vi "SubVI_SVM_train_Craik.vi"(4 "Max Passes":i32=15, 6 "C":dbl, 7 "Label Data":dbl[][](array[numeric]), 9 "Gamma":dbl, 10 "Linear or Gaussian":string, 11 "Training Data":dbl[][](array[numeric])) -> (0 "Alpha (idx)":dbl[][](array[numeric]), 1 "Label (idx)":dbl[][](array[numeric]), 2 "b":dbl, 3 "Training (idx)":dbl[][](array[numeric]), 5 "w":dbl[][](array[numeric]), 8 "Kernel Type":string)   [LabVIEW 2020]
uses:
  <vilib>/numeric/Random Number (Range) I64.vi
  <vilib>/Analysis/baseanly.llb/Real A x B.vi
  <vilib>/numeric/sub_Random U32.vi
  <vilib>/Analysis/Matrix/Numeric/Conversions/Matrix To Array - RM.vi
  <vilib>/Analysis/NI_AALBase.lvlib
  <vilib>/Analysis/Matrix/NI_Matrix.lvlib
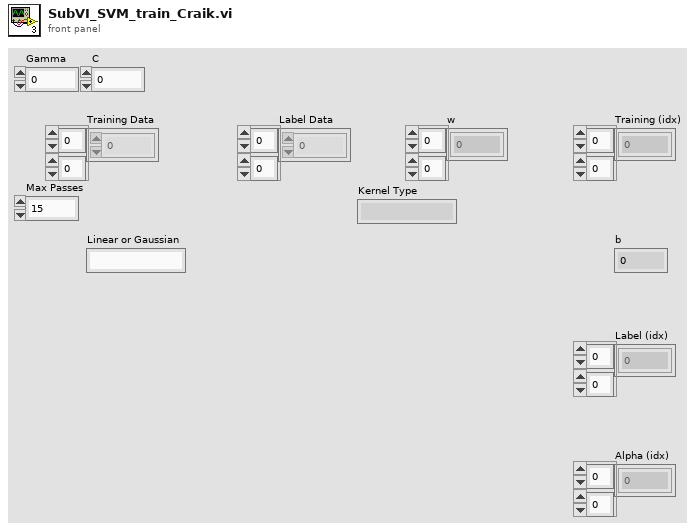
[diagram p1: front panel]
types:
  T1 = typedef "NI_Matrix.lvlib/RealMatrix.ctl" = dbl[][]
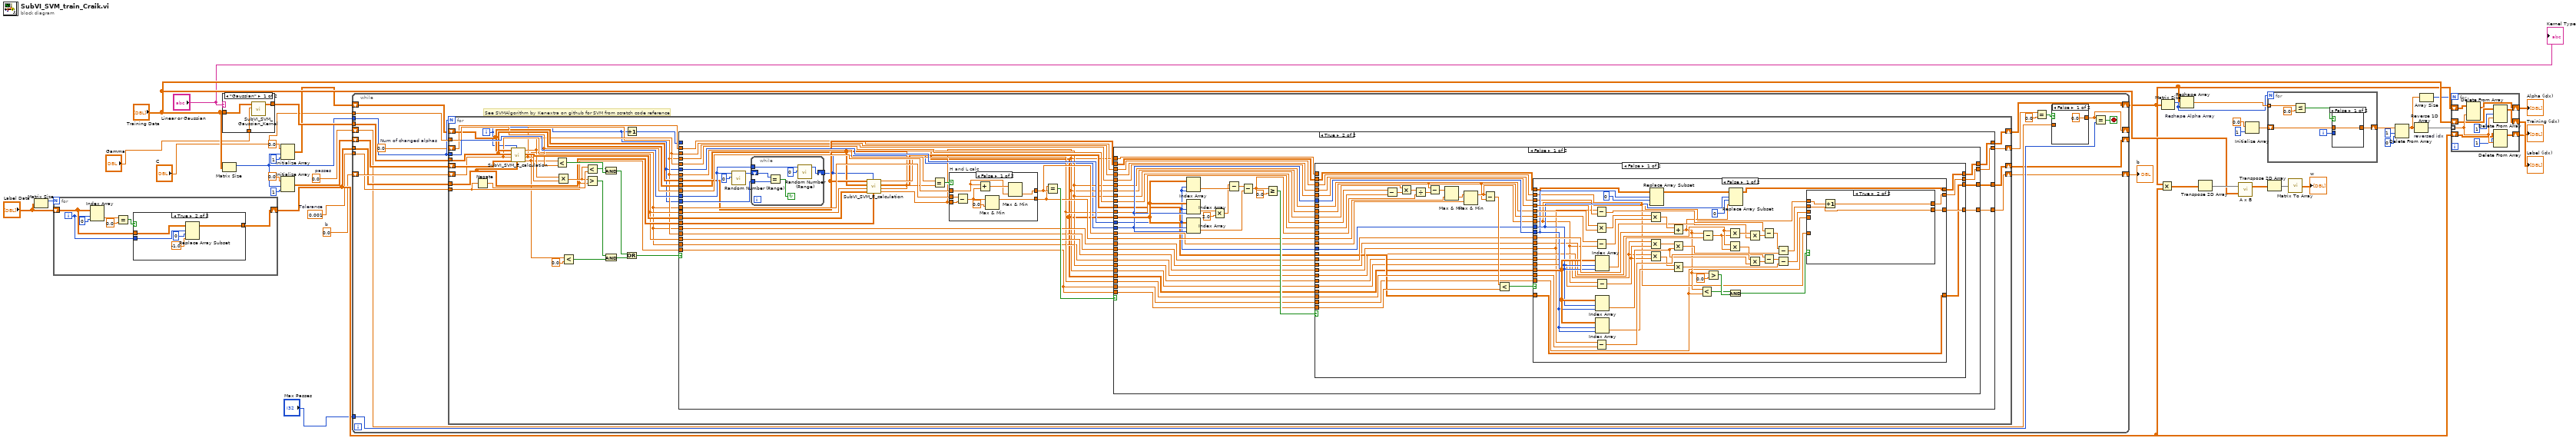
[diagram p0: block diagram]
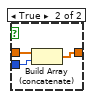
[diagram p2: hidden frame]
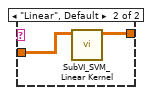
[diagram p3: hidden frame]
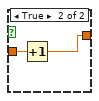
[diagram p4: hidden frame]
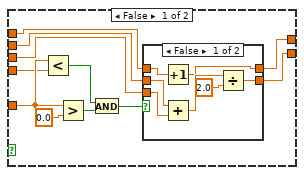
[diagram p6: hidden frame]
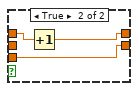
[diagram p7: hidden frame]
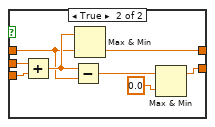
[diagram p11: hidden frame]
diagram:
  w4 = 0.001  # Tolerance
  w13 = 0.0  # passes
  w10 = 0.0  # b
  n1 = Matrix Size(0:"Label Data") -> (1:w5:i32)  [unwired: 1 out]
  n2 = for {
    N: w5 -> [_]
    shift-right: [w41] -> w40
    shift-left: "Label Data" -> [w43]
    i -> [w42]
    n3 = Index Array(array=w43, index (row)=w42, index (col)=0 ("disabled index (col)")) -> (element=w46:dbl)
    n4 = Equal?(x=w46, y=0.0) -> (x = y?=w47:bool)
    n5 = case shown="True" w47 {
      tunnel: w43 -> [w48 w53]
      tunnel: w42 -> [_ w52]
      tunnel: [w48 w49] -> w41
      frame False {
      }
      frame True {
        n6 = Replace Array Subset(array=w53, new element=-1.0 ("new element/subarray"), index (row)=w52, index (col)=0 ("disabled index (col)")) -> (w49:dbl[][])
      }
    }
  }
  n7 = case shown="\"Gaussian\"" "Linear or Gaussian" {
    tunnel: "Training Data" -> [w56 w58]
    tunnel: [w55 w57] -> w16
    tunnel: "Gamma" -> [w54 _]
    frame "Gaussian" {
      n8 = call "SubVI_SVM_Gaussian_Kernel.vi"("sigma"=w54, "X"=w56) -> ("K"=w55:dbl[][])  [unwired: 9 in]
    }
    frame "Linear", Default {
      n9 = call "SubVI_SVM_Linear Kernel.vi"("X"=w58) -> ("K"=w57:T1)  [unwired: 10 in]
    }
  }
  n10 = Matrix Size(0:"Training Data") -> (1:w12:i32)  [unwired: 1 out]
  n11 = Initialize Array(0.0 ("element"), w12, 1 ("dimension size")) -> (w14:dbl[][])
  n12 = Initialize Array(0.0 ("element"), w12, 1 ("dimension size")) -> (w11:dbl[][])
  n13 = while {
    tunnel: w40 -> [w76]
    tunnel: w4 -> [w74]
    tunnel: "C" -> [w73]
    tunnel: w12 -> [w72]
    shift-right: [w64] -> _
    shift-left: w13 -> [w66]
    tunnel: "Max Passes" -> [w63]
    shift-right: [w61] -> _
    shift-left: w11 -> [w75]
    tunnel: w16 -> [w70]
    shift-right: [w71] -> w32
    shift-left: w14 -> [w60]
    shift-right: [w59] -> w15
    shift-left: w10 -> [w77]
    stop <- w62 stop-if-true
    w69 = 0.0  # Num of changed alphas
    # "See SVMAlgorithm by Kenextra on github for SVM from scratch code reference"
    n14 = for {
      N: w72 -> [_]
      tunnel: w70 -> [w97]
      shift-right: [w91] -> w71
      shift-left: w60 -> [w92]
      tunnel: w76 -> [w95]
      shift-right: [w87] -> w61
      shift-left: w75 -> [w109]
      tunnel: w74 -> [w93]
      tunnel: w73 -> [w94]
      tunnel: w72 -> [w98]
      shift-right: [w89] -> w59
      shift-left: w77 -> [w90]
      shift-right: [w83] -> w68
      shift-left: w69 -> [w84]
      i -> [w82]
      n15 = Negate(x=w93) -> (-x=w108:dbl)
      n16 = call "SubVI_SVM_E_calculation.vi"("Y"=w95, "Index"=w82, "E"=w109, "b"=w90, "K"=w97, "Alphas"=w92) -> ("alpha[index]"=w85:dbl, "y[index]"=w86:dbl, "E"=w96:T1, "E[index]"=w88:dbl)  [unwired: 2 in]
      n17 = Less?(x=w85, y=w94) -> (x < y?=w107:bool)
      n18 = Multiply(x=w88, y=w86) -> (x*y=w105:dbl)
      n19 = Less?(x=w85, y=0.0) -> (x < y?=w102:bool)
      n20 = Less?(x=w105, y=w108) -> (x < y?=w106:bool)
      n21 = Greater?(x=w105, y=w93) -> (0:w104:bool)
      n22 = And(x=w106, y=w107) -> (x .and. y?=w100:bool)
      n23 = And(x=w104, y=w102) -> (x .and. y?=w101:bool)
      n24 = Or(x=w100, y=w101) -> (x .or. y?=w99:bool)
      n25 = Increment(x=w82) -> (x+1=w81:i32)
      n26 = case shown="True" w99 {
        tunnel: w98 -> [_ w146]
        tunnel: w82 -> [_ w147]
        tunnel: w92 -> [w113 w135]
        tunnel: w97 -> [_ w119]
        tunnel: w90 -> [_ w144]
        tunnel: w96 -> [w111 w143]
        tunnel: w95 -> [_ w142]
        tunnel: w86 -> [_ w141]
        tunnel: w85 -> [_ w139]
        tunnel: w94 -> [_ w138]
        tunnel: w82 -> [_ w136]
        tunnel: w88 -> [_ w134]
        tunnel: w93 -> [_ w118]
        tunnel: w85 -> [_ w131]
        tunnel: w86 -> [_ w130]
        tunnel: [w113 w129] -> w91
        tunnel: w90 -> [w112 w128]
        tunnel: [w112 w114] -> w89
        tunnel: w88 -> [_ w127]
        tunnel: [w111 w124] -> w87
        tunnel: w86 -> [_ w123]
        tunnel: w85 -> [_ w121]
        tunnel: w84 -> [w110 w117]
        tunnel: [w110 w116] -> w83
        tunnel: w81 -> [_ _]
        frame False {
        }
        frame True {
          n27 = call-poly <vilib>:"Random Number (Range).vi"("lower bound (-100)"=i64 0, "upper bound (100)"=w146) -> ("number"=w148:i64)  [unwired: 9 in]
          n28 = while {
            shift-right: [w330] -> w115
            shift-left: w148 -> [w334]
            tunnel: w147 -> [w333]
            tunnel: w146 -> [w331]
            stop <- w332 continue-if-true
            n29 = Equal?(x=w334, y=w333) -> (x = y?=w332:bool)
            n30 = call-poly <vilib>:"Random Number (Range).vi"("lower bound (-100)"=i64 0, "upper bound (100)"=w331) -> ("number"=w330:i64)  [unwired: 9 in]
          }
          n31 = call "SubVI_SVM_E_calculation.vi"("Y"=w142, "Index"=w115, "E"=w143, "b"=w144, "K"=w119, "Alphas"=w135) -> ("alpha[index]"=w120:dbl, "y[index]"=w122:dbl, "E"=w125:T1, "E[index]"=w126:dbl)  [unwired: 2 in]
          n32 = Equal?(x=w141, y=w122) -> (x = y?=w140:bool)
          n33 = case "H and L calc" shown="False" w140 {
            tunnel: w139 -> [w320 w328]
            tunnel: w120 -> [w319 w327]
            tunnel: w138 -> [w314 w322]
            tunnel: [w317 w324] -> w132
            tunnel: [w313 w321] -> w133
            frame False {
              n34 = Subtract(x=w320, y=w319) -> (x-y=w316:dbl)
              n35 = Add(x=w314, y=w316) -> (x+y=w315:dbl)
              n36 = Max & Min(x=w316, y=0.0) -> (max(x,y)=w317:dbl)  [unwired: 1 out]
              n37 = Max & Min(x=w315, y=w314) -> (min(x,y)=w313:dbl)  [unwired: 1 out]
            }
            frame True {
              n38 = Add(x=w328, y=w327) -> (x+y=w323:dbl)
              n39 = Subtract(x=w323, y=w322) -> (x-y=w326:dbl)
              n40 = Max & Min(x=w323, y=w322) -> (min(x,y)=w321:dbl)  [unwired: 1 out]
              n41 = Max & Min(x=w326, y=0.0) -> (max(x,y)=w324:dbl)  [unwired: 1 out]
            }
          }
          n42 = Equal?(x=w132, y=w133) -> (x = y?=w137:bool)
          n43 = case shown="False" w137 {
            tunnel: w119 -> [w187 _]
            tunnel: w136 -> [w168 _]
            tunnel: w115 -> [w180 _]
            tunnel: w135 -> [w181 w312]
            tunnel: w120 -> [w179 _]
            tunnel: w122 -> [w178 _]
            tunnel: w126 -> [w177 _]
            tunnel: w134 -> [w176 _]
            tunnel: w133 -> [w175 _]
            tunnel: w132 -> [w174 _]
            tunnel: w120 -> [w173 _]
            tunnel: w118 -> [w172 _]
            tunnel: w131 -> [w171 _]
            tunnel: w130 -> [w170 _]
            tunnel: w122 -> [w169 _]
            tunnel: [w167 w312] -> w129
            tunnel: w128 -> [w162 w311]
            tunnel: [w161 w311] -> w114
            tunnel: w127 -> [w160 _]
            tunnel: w126 -> [w159 _]
            tunnel: w125 -> [w158 w310]
            tunnel: [w157 w310] -> w124
            tunnel: w123 -> [w156 _]
            tunnel: w122 -> [w155 _]
            tunnel: w121 -> [w154 _]
            tunnel: w120 -> [w153 _]
            tunnel: w119 -> [w152 _]
            tunnel: w118 -> [w151 _]
            tunnel: w117 -> [w150 w309]
            tunnel: [w149 w309] -> w116
            frame False {
              n44 = Index Array(array=w187, index (row)=w168, index (col)=w168) -> (element=w186:dbl)
              n45 = Index Array(array=w187, index (row)=w168, index (col)=w180) -> (element=w166:dbl)
              n46 = Index Array(array=w187, index (row)=w180, index (col)=w180) -> (element=w184:dbl)
              n47 = Multiply(x=w166, y=2.0) -> (x*y=w164:dbl)
              n48 = Subtract(x=w164, y=w186) -> (x-y=w185:dbl)
              n49 = Subtract(x=w185, y=w184) -> (x-y=w163:dbl)
              n50 = Greater Or Equal?(x=w163, y=0.0) -> (x >= y?=w182:bool)
              n51 = case shown="False" w182 {
                tunnel: w181 -> [w224 w308]
                tunnel: w180 -> [w223 _]
                tunnel: w179 -> [_ _]
                tunnel: w178 -> [w220 _]
                tunnel: w177 -> [w221 _]
                tunnel: w176 -> [w222 _]
                tunnel: w163 -> [w217 _]
                tunnel: w175 -> [w216 _]
                tunnel: w174 -> [w214 _]
                tunnel: w173 -> [w204 _]
                tunnel: w172 -> [w212 _]
                tunnel: w171 -> [w209 _]
                tunnel: w170 -> [w208 _]
                tunnel: w169 -> [w207 _]
                tunnel: w168 -> [w206 _]
                tunnel: [w205 w308] -> w167
                tunnel: w162 -> [w201 w307]
                tunnel: [w200 w307] -> w161
                tunnel: w160 -> [w199 _]
                tunnel: w159 -> [w198 _]
                tunnel: w158 -> [w197 w306]
                tunnel: [w196 w306] -> w157
                tunnel: w156 -> [w195 _]
                tunnel: w155 -> [w194 _]
                tunnel: w154 -> [w193 _]
                tunnel: w153 -> [w192 _]
                tunnel: w152 -> [w191 _]
                tunnel: w151 -> [w190 _]
                tunnel: w150 -> [w189 w305]
                tunnel: [w188 w305] -> w149
                frame False {
                  n52 = Subtract(x=w222, y=w221) -> (x-y=w219:dbl)
                  n53 = Multiply(x=w220, y=w219) -> (x*y=w218:dbl)
                  n54 = Divide(x=w218, y=w217) -> (x/y=w203:dbl)
                  n55 = Subtract(x=w204, y=w203) -> (x-y=w202:dbl)
                  n56 = Max & Min(x=w202, y=w216) -> (min(x,y)=w215:dbl)  [unwired: 1 out]
                  n57 = Max & Min(x=w215, y=w214) -> (max(x,y)=w210:dbl)  [unwired: 1 out]
                  n58 = Subtract(x=w210, y=w204) -> (x-y=w213:dbl)
                  n59 = Less?(x=w213, y=w212) -> (x < y?=w211:bool)
                  n60 = case shown="False" w211 {
                    tunnel: w224 -> [w276 w304]
                    tunnel: w223 -> [w261 _]
                    tunnel: [w272 w304] -> w205
                    tunnel: w210 -> [w229 _]
                    tunnel: w209 -> [w266 _]
                    tunnel: w204 -> [w274 _]
                    tunnel: w208 -> [w270 _]
                    tunnel: w207 -> [w269 _]
                    tunnel: w206 -> [w262 _]
                    tunnel: w201 -> [w244 w303]
                    tunnel: [w230 w303] -> w200
                    tunnel: w199 -> [w257 _]
                    tunnel: w198 -> [w243 _]
                    tunnel: [w264 w302] -> w196
                    tunnel: w197 -> [w264 w302]
                    tunnel: w195 -> [w242 _]
                    tunnel: w194 -> [w238 _]
                    tunnel: w193 -> [w260 _]
                    tunnel: w192 -> [w254 _]
                    tunnel: w191 -> [w263 _]
                    tunnel: w190 -> [w227 _]
                    tunnel: w189 -> [w226 w301]
                    tunnel: [w225 w301] -> w188
                    frame False {
                      n61 = Subtract(x=w244, y=w257) -> (x-y=w256:dbl)
                      n62 = Multiply(x=w270, y=w269) -> (x*y=w267:dbl)
                      n63 = Subtract(x=w274, y=w229) -> (x-y=w268:dbl)
                      n64 = Subtract(x=w244, y=w243) -> (x-y=w249:dbl)
                      n65 = Subtract(x=w229, y=w254) -> (x-y=w239:dbl)
                      n66 = Index Array(array=w263, index (row)=w262, index (col)=w262) -> (element=w258:dbl)
                      n67 = Index Array(array=w263, index (row)=w262, index (col)=w261) -> (element=w240:dbl)
                      n68 = Index Array(array=w263, index (row)=w261, index (col)=w261) -> (element=w237:dbl)
                      n69 = Multiply(x=w267, y=w268) -> (x*y=w265:dbl)
                      n70 = Multiply(x=w238, y=w239) -> (x*y=w253:dbl)
                      n71 = Multiply(x=w238, y=w239) -> (x*y=w247:dbl)
                      n72 = Replace Array Subset(array=w276, new element=w229, index (row)=w261, index (col)=0 ("disabled index (col)")) -> (w273:dbl[][])
                      n73 = Add(x=w265, y=w266) -> (x+y=w235:dbl)
                      n74 = Multiply(x=w253, y=w240) -> (x*y=w251:dbl)
                      n75 = Multiply(x=w247, y=w237) -> (x*y=w245:dbl)
                      n76 = Less?(x=w235, y=w227) -> (x < y?=w233:bool)
                      n77 = Subtract(x=w235, y=w260) -> (x-y=w241:dbl)
                      n78 = Greater?(x=w235, y=0.0) -> (0:w234:bool)
                      n79 = Multiply(x=w242, y=w241) -> (x*y=w259:dbl)
                      n80 = Multiply(x=w242, y=w241) -> (x*y=w250:dbl)
                      n81 = And(x=w233, y=w234) -> (x .and. y?=w232:bool)
                      n82 = Replace Array Subset(array=w273, new element=w235, index (row)=w262, index (col)=0 ("disabled index (col)")) -> (w272:dbl[][])
                      n83 = Multiply(x=w259, y=w258) -> (x*y=w255:dbl)
                      n84 = Multiply(x=w250, y=w240) -> (x*y=w248:dbl)
                      n85 = Subtract(x=w256, y=w255) -> (x-y=w252:dbl)
                      n86 = Subtract(x=w249, y=w248) -> (x-y=w246:dbl)
                      n87 = Subtract(x=w252, y=w251) -> (x-y=w231:dbl)
                      n88 = Subtract(x=w246, y=w245) -> (x-y=w228:dbl)
                      n89 = case shown="True" w232 {
                        tunnel: w231 -> [w280 w300]
                        tunnel: [w281 w300] -> w230
                        tunnel: w229 -> [w284 _]
                        tunnel: w228 -> [w282 _]
                        tunnel: w227 -> [w279 _]
                        tunnel: w226 -> [w278 w299]
                        tunnel: [w277 w298] -> w225
                        frame False {
                          n90 = Less?(x=w284, y=w279) -> (x < y?=w285:bool)
                          n91 = Greater?(x=w284, y=0.0) -> (0:w286:bool)
                          n92 = And(x=w285, y=w286) -> (x .and. y?=w283:bool)
                          n93 = case shown="False" w283 {
                            tunnel: w282 -> [w293 w297]
                            tunnel: [w290 w297] -> w281
                            tunnel: w280 -> [w294 _]
                            tunnel: w278 -> [w289 w296]
                            tunnel: [w288 w295] -> w277
                            frame False {
                              n94 = Increment(x=w289) -> (x+1=w288:dbl)
                              n95 = Add(x=w294, y=w293) -> (x+y=w292:dbl)
                              n96 = Divide(x=w292, y=2.0) -> (x/y=w290:dbl)
                            }
                            frame True {
                              n97 = Increment(x=w296) -> (x+1=w295:dbl)
                            }
                          }
                        }
                        frame True {
                          n98 = Increment(x=w299) -> (x+1=w298:dbl)
                        }
                      }
                    }
                    frame True {
                    }
                  }
                }
                frame True {
                }
              }
            }
            frame True {
            }
          }
        }
      }
    }
    n99 = Equal?(x=w68, y=0.0) -> (x = y?=w65:bool)
    n100 = case shown="False" w65 {
      tunnel: w66 -> [_ w80]
      tunnel: [0.0 w79] -> w64
      frame False {
      }
      frame True {
        n101 = Increment(x=w80) -> (x+1=w79:dbl)
      }
    }
    n102 = Equal?(x=w64, y=w63) -> (x = y?=w62:bool)
  }
  "b" <- w15
  n103 = Multiply(x=w32, y=w40) -> (x*y=w34:dbl[][])
  n104 = Matrix Size(0:w32) -> (1:w25:i32)  [unwired: 1 out]
  n105 = Reshape Array "Reshape Alpha Array"(w32, w25) -> (w26:dbl[])
  n106 = Transpose 2D Array(2D array=w34) -> (transposed array=w35:dbl[][])
  n107 = call-poly <vilib>:"A x B.vi"("B"="Training Data", "A"=w35) -> ("A x B"=w36:T1)  [unwired: 1 out]
  n108 = Initialize Array(0.0 ("element"), 1 ("dimension size")) -> (w20:dbl[])
  n109 = for {
    N: w25 -> [_]
    tunnel: w26 -> [w340] mode=indexing
    shift-right: [w335] -> w21
    shift-left: w20 -> [w337]
    i -> [w336]
    n110 = Less Or Equal?(x=w340, y=0.0) -> (x <= y?=w338:bool)
    n111 = case shown="False" w338 {
      tunnel: w337 -> [w341 w344]
      tunnel: w336 -> [_ w343]
      tunnel: [w341 w342] -> w335
      frame False {
      }
      frame True {
        n112 = Build Array (concatenate)(w344, w343) -> (w342:dbl[])
      }
    }
  }
  n113 = Transpose 2D Array(2D array=w36) -> (transposed array=w37:T1)
  n114 = call-poly <vilib>:"Matrix To Array.vi"("Real Matrix"=w37) -> ("Real 2D Array"=→"w":dbl[][])
  n115 = Delete From Array(array=w21, length=1, index=0) -> (array with subset deleted=w27:dbl[])  [unwired: 1 out]
  n116 = Reverse 1D Array "reversed idx"(array=w27) -> (reversed array=w28:dbl[])
  n117 = Array Size(array=w27) -> (size(s)=w24:i32)
  n118 = for {
    N: w24 -> [_]
    tunnel: w28 -> [w353] mode=indexing
    shift-right: [w351] -> w29
    shift-left: w40 -> [w352]
    shift-right: [w347] -> w30
    shift-left: "Training Data" -> [w348]
    shift-right: [w345] -> w31
    shift-left: w32 -> [w346]
    n119 = Delete From Array(array=w346, index (row)=w353) -> (array with subset deleted=w345:dbl[][])  [unwired: 2 in, 1 out]
    n120 = Delete From Array(array=w348, length=1, index (row)=w353) -> (array with subset deleted=w347:dbl[][])  [unwired: 1 in, 1 out]
    n121 = Delete From Array(array=w352, length=1, index (row)=w353) -> (array with subset deleted=w351:dbl[][])  [unwired: 1 in, 1 out]
  }
  "Alpha (idx)" <- w31
  "Training (idx)" <- w30
  "Label (idx)" <- w29
  "Kernel Type" <- "Linear or Gaussian"
